vi "calculateNumber.vi"(10 "Array":dbl[](array[numeric])) -> (2 "Number":dbl)   [LabVIEW 2013]
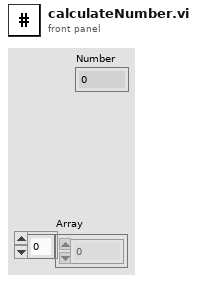
[diagram p1: front panel]
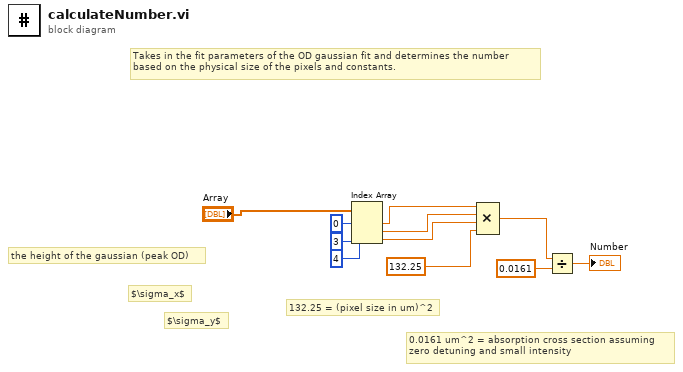
[diagram p0: block diagram]
diagram:
  # "Takes in the fit parameters of the OD gaussian fit and determines the number\nbased on the physical size of the pixels and constants."
  # "0.0161 um^2 = absorption cross section assuming\nzero detuning and small intensity"
  # "132.25 = (pixel size in um)^2"
  # "$\\sigma_y$"
  # "$\\sigma_x$"
  # "the height of the gaussian (peak OD)"
  n1 = Index Array(array="Array", index #1=0 ("index"), index #2=3 ("index"), index #3=4 ("index")) -> (element #1=w5:dbl, element #2=w4:dbl, element #3=w3:dbl)
  n2 = Compound Arithmetic op=MULTIPLY(w5, w4, w3, 132.25 ("x")) -> (w1:dbl)
  n3 = Divide(x=w1, y=0.0161) -> (x/y=→"Number":dbl)
